vi "load_config.vi"(4 "error in (no error)":errorcluster, 5 "py interface file":path, 6 "Request data":variant, 7 "Python session in":refnum<k35>) -> (0 "error out":errorcluster, 2 "Response data":variant, 3 "Python session out":refnum<k35>)   [LabVIEW 2022 SP3]
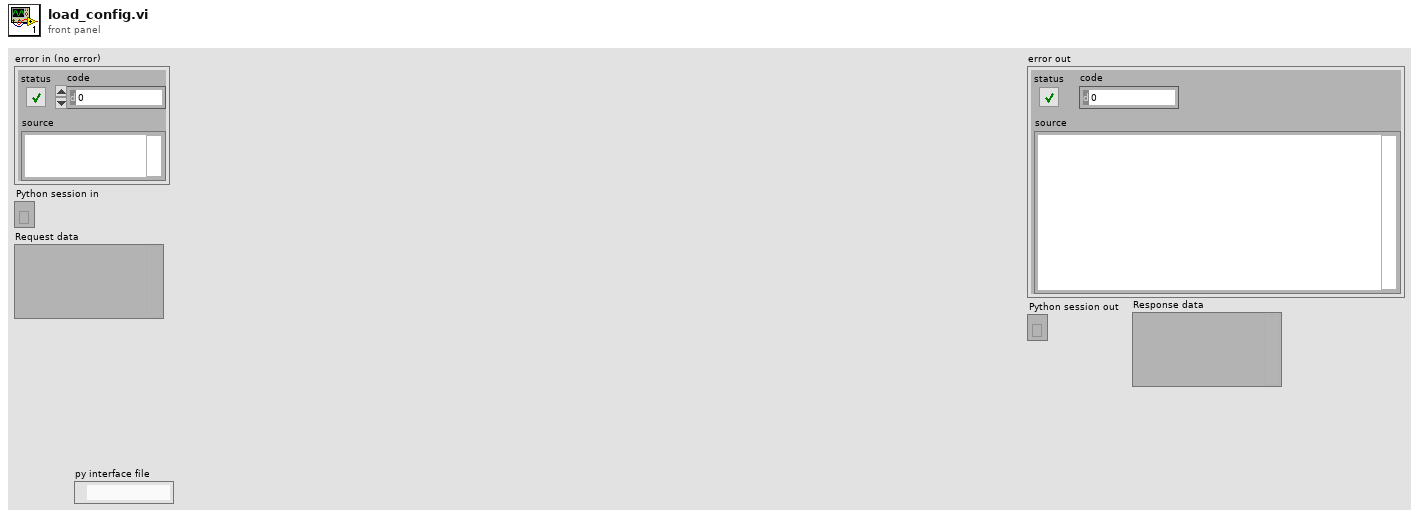
[diagram p1: front panel]
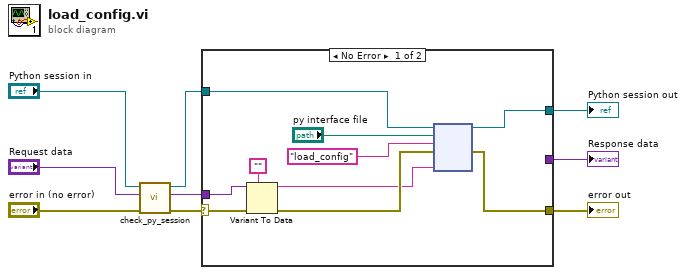
[diagram p0: block diagram]
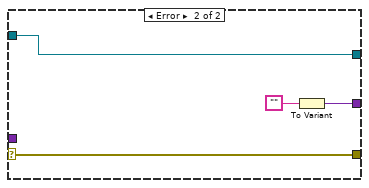
[diagram p2: hidden frame]
diagram:
  n1 = call "check_py_session.vi"("error in"="error in (no error)", "Request data"="Request data", "Python session in"="Python session in") -> ("error out"=w3:errorcluster, "Response data"=w4:variant, "Python session out"=w5:refnum<k35>)  [unwired: 2 in]
  n2 = case shown="No Error" w3 {
    selector: w3 -> [w18 w23]
    tunnel: w5 -> [w16 w22]
    tunnel: [w11 w22] -> w9
    tunnel: w4 -> [w19 _]
    tunnel: [w12 w23] -> w2
    tunnel: [_ w20] -> w1
    frame No Error {
      n3 = Variant To Data(error in=w18, type="", Variant=w19) -> (data=w10:string, error out=w13:errorcluster)
      n4 = node(w16, "py interface file", "load_config" ("function name"), w13, w10) -> (w11:refnum<k35>, w12:errorcluster)  [unwired: 3 in, 2 out]
    }
    frame Error {
      n5 = To Variant(anything="") -> (Variant=w20:variant)
    }
  }
  "error out" <- w2
  "Python session out" <- w9
  "Response data" <- w1
